vi "Import.vi"(8 "error in":errorcluster, 11 "CSV Path":path=path "C:/Users/Administrator/Desktop/FPGA Wizard/Exported IO.csv") -> (0 "error out":errorcluster, 3 "FPGA Settings":T1[](array[typedef]))   [LabVIEW 2015, in "Project.lvclass"]
uses:
  Project.lvclass
  FPGA Settings.ctl
  Module/Module/Module Settings.ctl
  Signal/Signal/Signal Settings.ctl
  Signal/Signal/Signal.lvclass
  Module/Module/Module.lvclass
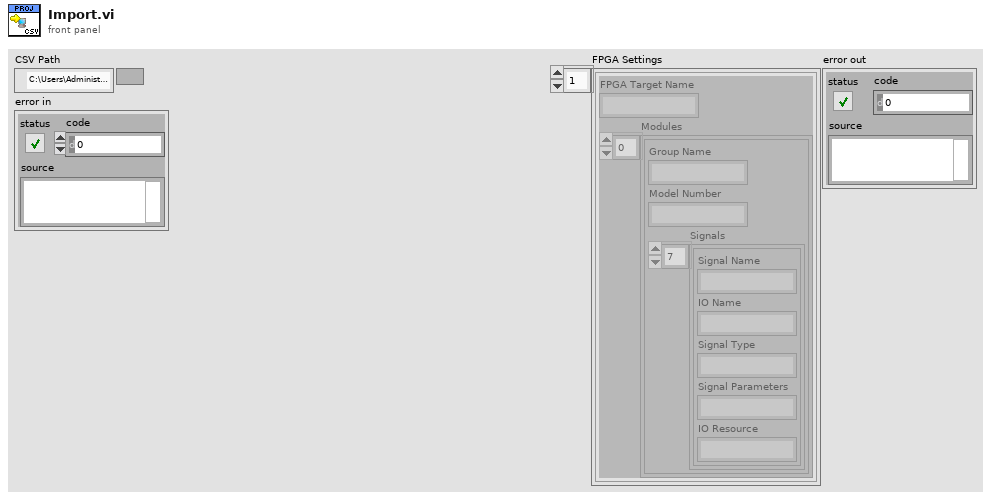
[diagram p1: front panel]
types:
  T1 = typedef "Project.lvclass/FPGA Settings.ctl" = cluster{"FPGA Target Name":string, "Modules":T2[]}
  T2 = typedef "Module.lvclass/Module Settings.ctl" = cluster{"Group Name":string, "Model Number":string, "Signals":T3[]}
  T3 = typedef "Signal.lvclass/Signal Settings.ctl" = cluster{"Signal Name":string, "IO Name":string, "Signal Type":string, "Signal Parameters":string, "IO Resource":string}
  T4 = enum16{"open", "replace", "create", "open or create", "replace or create", "replace or create with confirmation"}
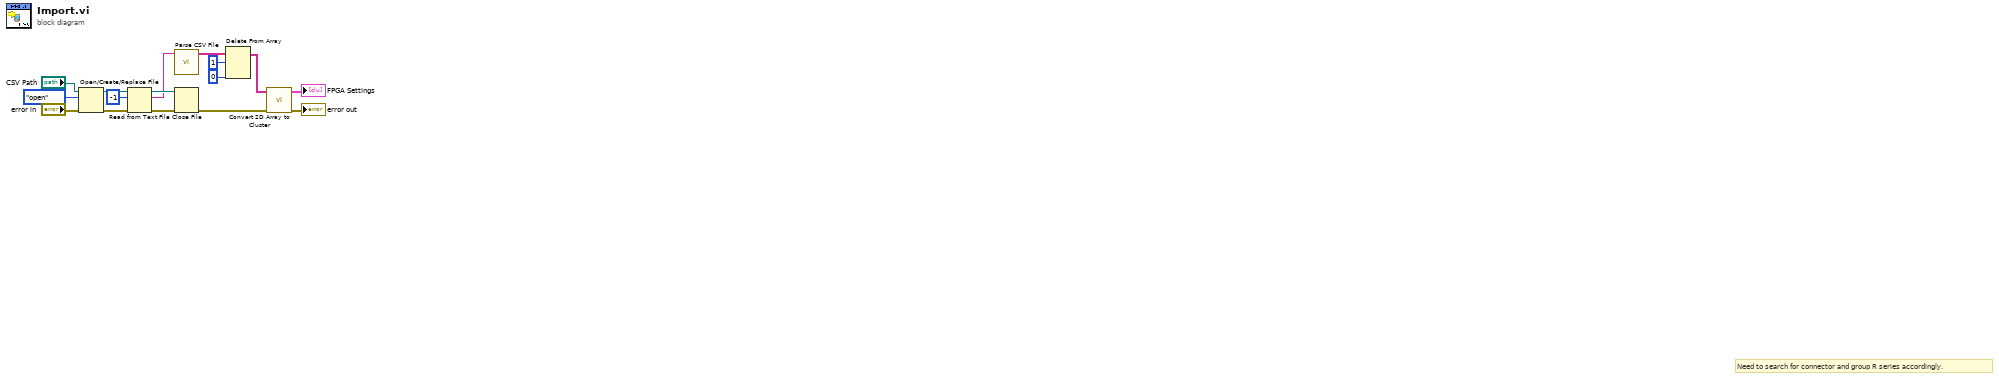
[diagram p0: block diagram]
diagram:
  # "Need to search for connector and group R series accordingly."
  n1 = Open/Create/Replace File(file path (use dialog)="CSV Path", error in="error in", operation (0:open)=T4."open") -> (refnum out=w16:refnum<file>, error out=w13:errorcluster)  [unwired: 3 in, 1 out]
  n2 = Read from Text File(file (use dialog)=w16, count=-1, error in=w13) -> (refnum out=w15:refnum<file>, text=w3:string, error out=w14:errorcluster)  [unwired: 1 in, 1 out]
  n3 = call "Parse CSV File.vi"("String"=w3) -> ("Array"=w2:string[][])  [unwired: 10 in]
  n4 = Close File(refnum=w15, error in=w14) -> (error out=w6:errorcluster)  [unwired: 1 out]
  n5 = Delete From Array(array=w2, length=1, index (row)=0) -> (array with subset deleted=w9:string[][])  [unwired: 1 in, 1 out]
  n6 = call "Convert 2D Array to Cluster.vi"("error in (no error)"=w6, "Array in"=w9) -> ("error out"=→"error out":errorcluster, "Array out"=→"FPGA Settings":T1[])  [unwired: 8 in]
